vi "计算V2实际电压.vi"(11 "数值":dbl) -> (3 "x/y":dbl format="%_8g")   [LabVIEW 2018]
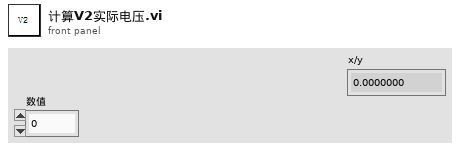
[diagram p1: front panel]
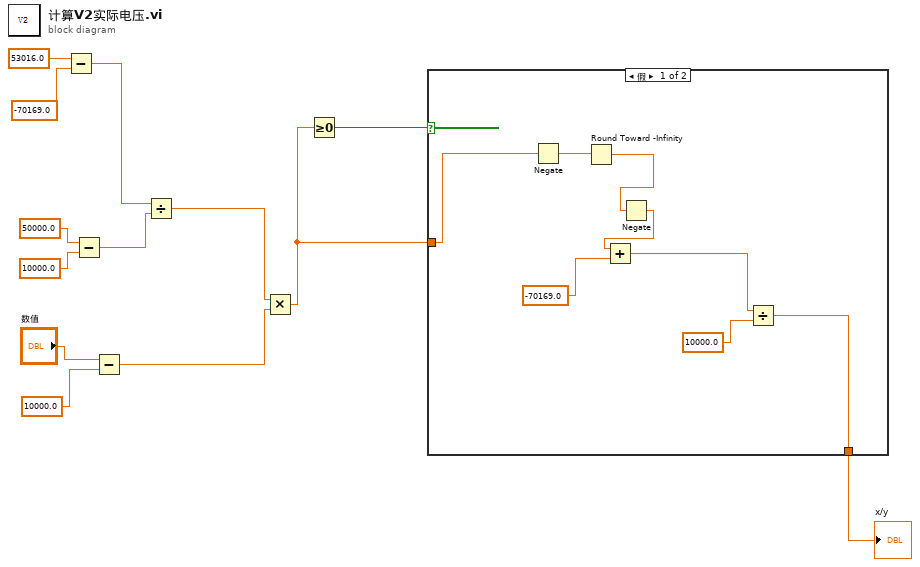
[diagram p0: block diagram]
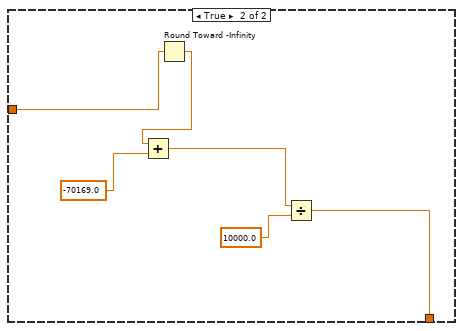
[diagram p2: hidden frame]
diagram:
  n1 = Subtract(x=53016.0, y=-70169.0) -> (x-y=w13:dbl)
  n2 = Subtract(x=50000.0, y=10000.0) -> (x-y=w12:dbl)
  n3 = Subtract(x="数值", y=10000.0) -> (x-y=w10:dbl)
  n4 = Divide(x=w13, y=w12) -> (x/y=w9:dbl)
  n5 = Multiply(x=w9, y=w10) -> (x*y=w2:dbl)
  n6 = Greater Or Equal To 0?(x=w2) -> (x >= 0?=w3:bool)
  n7 = case shown="假" w3 {
    tunnel: w2 -> [w18 w27]
    tunnel: [w14 w22] -> w1
    frame False {
      n8 = Negate(x=w18) -> (-x=w17:dbl)
      n9 = Round Toward -Infinity(1:w17) -> (0:w16:dbl)
      n10 = Negate(x=w16) -> (-x=w15:dbl)
      n11 = Add(x=w15, y=-70169.0) -> (x+y=w21:dbl)
      n12 = Divide(x=w21, y=10000.0) -> (x/y=w14:dbl)
    }
    frame True {
      n13 = Round Toward -Infinity(1:w27) -> (0:w23:dbl)
      n14 = Add(x=w23, y=-70169.0) -> (x+y=w26:dbl)
      n15 = Divide(x=w26, y=10000.0) -> (x/y=w22:dbl)
    }
  }
  "x/y" <- w1
